vi "Write Update Events.vi"(8 "error in (no error)":errorcluster, 10 "Update Events":T1, 11 "CS++Nanotec in":refnum<class "CS++Nanotec.lvclass">) -> (0 "error out":errorcluster, 3 "CS++Nanotec out":refnum<class "CS++Nanotec.lvclass">)   [LabVIEW 2015, in "CS++Nanotec.lvlib" / "CS++Nanotec.lvclass"]
uses:
  CS++Nanotec.lvclass
  CS++Nanotec.lvclass/CS++Nanotec.ctl
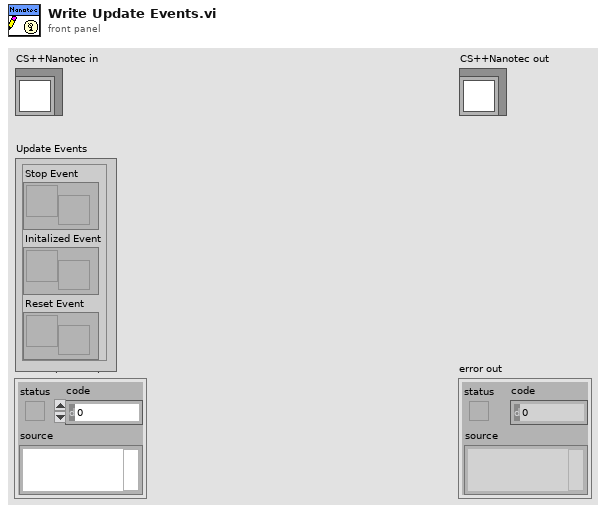
[diagram p1: front panel]
types:
  T1 = cluster{"Stop Event":refnum<user-event>, "Initalized Event":refnum<user-event>, "Reset Event":refnum<user-event>}
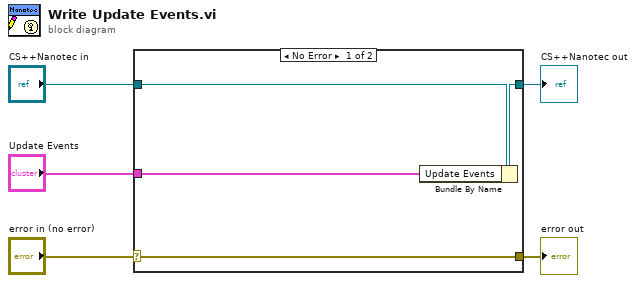
[diagram p0: block diagram]
diagram:
  n1 = case shown="No Error" "error in (no error)" {
    selector: "error in (no error)" -> [w9 w10]
    tunnel: [w9 w10] -> w4
    tunnel: [w7 w11] -> w2
    tunnel: "CS++Nanotec in" -> [w8 w11]
    tunnel: "Update Events" -> [w6 _]
    frame No Error {
      n2 = Bundle By Name(cluster=w8, "Update Events"=w6) -> (w7:refnum<class "CS++Nanotec.lvclass">)
    }
    frame Error {
    }
  }
  "error out" <- w4
  "CS++Nanotec out" <- w2
